vi "Open Serial.vi"(4 "Timeout":u32, 5 "Stop Bits":u8, 6 "Parity":T1, 7 "Data Bits":u8, 8 "error in (no error)":errorcluster, 9 "Baudrate":u32, 10 "Serial Port":string) -> (0 "error out":errorcluster, 1 "baudrate":u32, 2 "Device Name":string, 3 "LINX Client out":refnum<class "LINX Client.lvclass">)   [LabVIEW 2020, in "LINX Client.lvclass"]
uses:
  LINX Client.lvclass
  Typedef/Parity.ctl
  LINX Base.lvclass
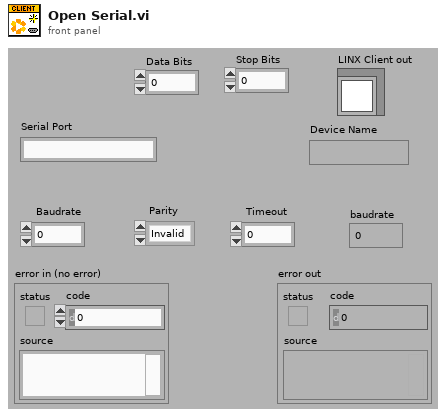
[diagram p1: front panel]
types:
  T1 = typedef "LINX Base.lvclass/Parity.ctl" = enum8{"Invalid", "None", "Odd", "Even", "Mark", "Space"}
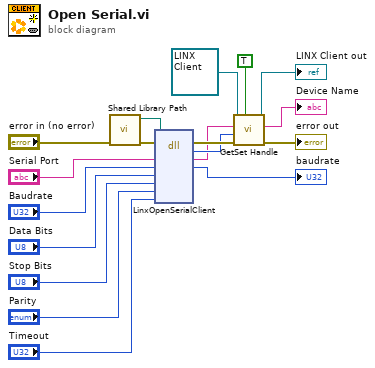
[diagram p0: block diagram]
diagram:
  n1 = call "Shared Library Path.vi"("error in (no error)"="error in (no error)") -> ("error out"=w16:errorcluster, "Path"=w18:path)  [unwired: 9 out]
  n2 = dll-call lib="Z:/Development/LabVIEW Hobbyist Toolkit/LabVIEW/vi.lib/MakerHub/LINX/Resources/libLinxDevice.dll" fn="LinxOpenSerialClient"(path in=w18, error in=w16, "name"="Serial Port", "baudrate"="Baudrate", "dataBits"="Data Bits", "stopBits"="Stop Bits", "parity"="Parity", "timeout"="Timeout") -> (error out=w8:errorcluster, "LinxDevice"=w6:u64, "name"=w3:string, "baudrate"=→"baudrate":u32)  [unwired: 4 in, 2 out]
  n3 = call-dynamic "GetSet Handle.vi"("store (F)"=TRUE, "error in"=w8, "handle in"=w6, "connection"=w3, "LINX Base in"=refnum<class "LINX Client.lvclass"> refnum ("LINX Device")) -> ("error out"=→"error out":errorcluster, "name"=→"Device Name":string, "LINX Base out"=→"LINX Client out":refnum<class "LINX Client.lvclass">)  [unwired: 1 in, 3 out]
